vi "asdk Send Pattern.vi"(7 "nRepeat":u32, 8 "error in (no error)":errorcluster, 9 "nPattern":u32, 11 "pDm":u64) -> (0 "error out":errorcluster, 3 "pDm out":u64)   [LabVIEW 2020, in "ASDK.lvlib"]
doc: "ASDK_API COMPL_STAT asdkSendPattern( asdkDM *pDm, const Scalar *pattern, UInt nPattern, UInt nRepeat );"
uses:
  ASDK.lvlib
  ASDK.dll
panel:
  in  "pattern":dbl[](array[numeric])
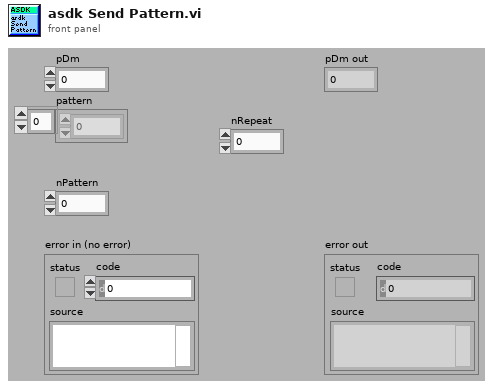
[diagram p1: front panel]
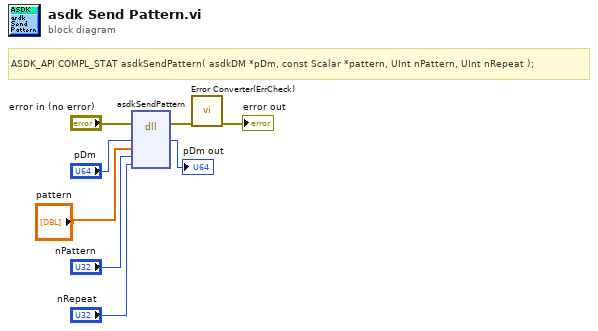
[diagram p0: block diagram]
diagram:
  # "ASDK_API COMPL_STAT asdkSendPattern( asdkDM *pDm, const Scalar *pattern, UInt nPattern, UInt nRepeat );"
  n1 = dll-call lib="ASDK.*" fn="asdkSendPattern"(error in="error in (no error)", "pDm"="pDm", "pattern"="pattern", "nPattern"="nPattern", "nRepeat"="nRepeat") -> (error out=w3:errorcluster, "pDm"=→"pDm out":u64)  [unwired: 6 in, 1 out]
  n2 = call "Error Converter(ErrCheck).vi"("error in (no error)"=w3) -> ("error out"=→"error out":errorcluster)  [unwired: 10 in]
